vi "GETDAcc.vi"(8 "error in (no error)":errorcluster, 11 "Tapedrive_ESP301 in":refnum<class "Tapedrive_ESP301.lvclass">) -> (0 "error out":errorcluster, 3 "Tapedrive_ESP301 out":refnum<class "Tapedrive_ESP301.lvclass">)   [LabVIEW 2013, in "Tapedrive_ESP301.lvclass"]
uses:
  Tapedrive_ESP301.lvclass
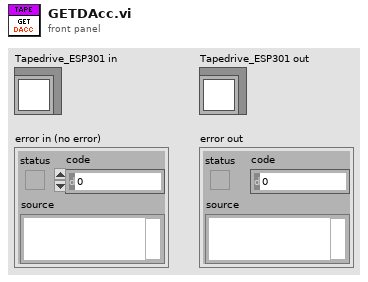
[diagram p1: front panel]
types:
  T1 = cluster{"Axis 1":cluster{"Value":dbl, "Min":dbl, "Max":dbl, "StepSize":dbl, "Tolerance":dbl, "ValueActual":dbl}, "Axis 2":cluster{"Value":dbl, "Min":dbl, "Max":dbl, "StepSize":dbl, "Tolerance":dbl, "ValueActual":dbl}}
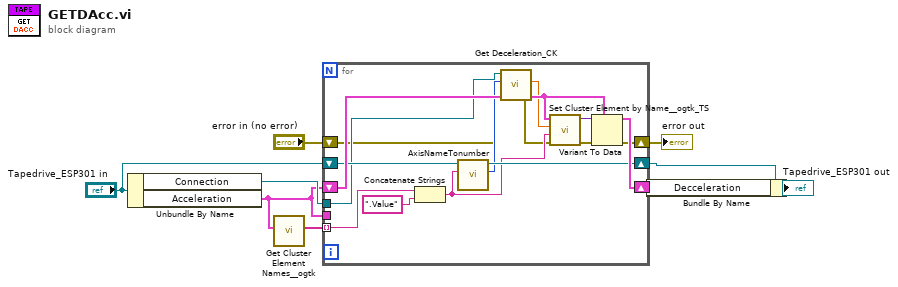
[diagram p0: block diagram]
diagram:
  n1 = Unbundle By Name("Tapedrive_ESP301 in") -> ("Connection"=w5:refnum<visa-resource-name>, "Acceleration"=w1:T1)
  n2 = call <userlib>:"Get Cluster Element Names__ogtk.vi"("Cluster"=w1) -> ("Element Names"=w2:string[])  [unwired: 9 in, 1 out]
  n3 = for {
    tunnel: w2 -> [w16] mode=indexing
    tunnel: w1 -> [_]
    shift-right: [w20] -> w3
    shift-left: w1 -> [w21]
    shift-right: [w18] -> w8
    shift-left: "Tapedrive_ESP301 in" -> [w19]
    tunnel: w5 -> [w14]
    shift-right: [w17] -> w7
    shift-left: "error in (no error)" -> [w11]
    n4 = Concatenate Strings(w16, ".Value" ("string")) -> (w15:string)
    n5 = call "AxisNameTonumber.vi"("Channel"=w15, "Tapedrive_ESP301 in"=w19) -> ("Axis No."=w13:i16, "Tapedrive_ESP301 out"=w18:refnum<class "Tapedrive_ESP301.lvclass">)  [unwired: 8 in]
    n6 = call "Get Deceleration_CK.vi"("error in (no error)"=w11, "Axis (1)"=w13, "VISA resource name"=w14) -> ("error out"=w10:errorcluster, "Deceleration (units/s²)"=w12:dbl)  [unwired: 2 in, 1 out]
    n7 = call "Set Cluster Element by Name__ogtk_TS.vi"("error in (no error)"=w10, "Element Name (\"\": New Element Data Name)"=w15, "New Element Value"=w12, "Cluster"=w21) -> ("error out"=w23:errorcluster, "VCluster out"=w22:variant)  [unwired: 5 in, 1 out]
    n8 = Variant To Data(error in=w23, type=w21, Variant=w22) -> (data=w20:T1, error out=w17:errorcluster)
  }
  "error out" <- w7
  n9 = Bundle By Name(cluster=w8, "Decceleration"=w3) -> (→"Tapedrive_ESP301 out":refnum<class "Tapedrive_ESP301.lvclass">)
